vi "Init.vi"(8 "error in":errorcluster, 10 "File Path":path, 11 "TDMS in":refnum<class "TDMS.lvclass">) -> (0 "error out":errorcluster, 3 "TDMS out":refnum<class "TDMS.lvclass">)   [LabVIEW 2017, in "Report_lib.lvlib" / "TDMS.lvclass"]
uses:
  TDMS.lvclass
  I:/TEMP/Source/Classes/Log/Log.lvclass
  Log/Log.lvclass/Log.ctl
  TDMS.lvclass/TDMS.ctl
  Log/Log.lvclass
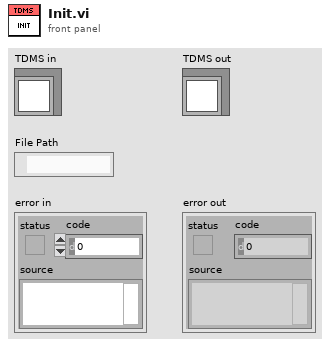
[diagram p1: front panel]
types:
  T1 = typedef "Log Data.ctl" = cluster{"File Path":path, "File Name":string, "File Ext":string}
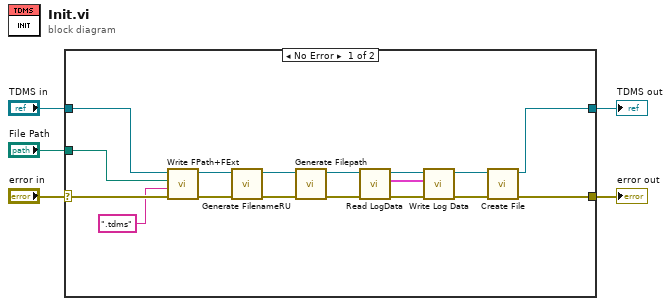
[diagram p0: block diagram]
diagram:
  n1 = case shown="No Error" "error in" {
    selector: "error in" -> [w22 w24]
    tunnel: [w12 w24] -> w4
    tunnel: [w13 w23] -> w2
    tunnel: "TDMS in" -> [w14 w23]
    tunnel: "File Path" -> [w10 _]
    frame No Error {
      n2 = call "Write FPath+FExt.vi"("error in (no error)"=w22, "File Ext"=".tdms", "File Path"=w10, "Log in"=w14) -> ("error out"=w8:errorcluster, "Log out"=w9:refnum<class "TDMS.lvclass">)  [unwired: 6 in]
      n3 = call "Generate FilenameRU.vi"("error in"=w8, "Log in"=w9) -> ("error out"=w6:errorcluster, "Log out"=w7:refnum<class "TDMS.lvclass">)  [unwired: 8 in]
      n4 = call "Generate Filepath.vi"("error in"=w6, "Log in"=w7) -> ("error out"=w20:errorcluster, "Log out"=w21:refnum<class "TDMS.lvclass">)  [unwired: 8 in]
      n5 = call "Read LogData.vi"("error in (no error)"=w20, "Log in"=w21) -> ("error out"=w17:errorcluster, "Log Data"=w18:T1, "Log out"=w19:refnum<class "TDMS.lvclass">)  [unwired: 7 in]
      n6 = call "Write Log Data.vi"("error in"=w17, "Log Data"=w18, "TDMS in"=w19) -> ("error out"=w15:errorcluster, "TDMS out"=w16:refnum<class "TDMS.lvclass">)  [unwired: 7 in]
      n7 = call-dynamic "Create File.vi"("error in"=w15, "TDMS in"=w16) -> ("error out"=w12:errorcluster, "TDMS out"=w13:refnum<class "TDMS.lvclass">)  [unwired: 8 in]
    }
    frame Error {
    }
  }
  "error out" <- w4
  "TDMS out" <- w2
